vi "DSF.Engine.Transfer.Set Channel Blocks.vi"(10 "Block Descriptors":T1[](array[typedef]) {"count" format="%d elements"; "First Channel Descriptor"."base address" format="%016x"; "First Channel Descriptor"."Channel Parameters"."offset" format="%d bytes"}, 11 "Transfer in":refnum<class "DSF.Engine.Transfer.lvclass">) -> (3 "Transfer out":refnum<class "DSF.Engine.Transfer.lvclass">)   [LabVIEW 2017, in "DSF.Engine.lvlib" / "DSF.Engine.Transfer.lvclass"]
uses:
  DSF.Engine.Transfer.lvclass
  Shared/Typedefs/DSF.Shared.Typedefs.Configuration.Transfer.Channel Block Descriptor.ctl
  Shared/Typedefs/DSF.Shared.Typedefs.Configuration.Transfer.Channel Descriptor.ctl
  Shared/Typedefs/DSF.Shared.Typedefs.Configuration.Transfer.Channel Parameters.ctl
  Shared/Typedefs/DSF.Shared.Typedefs.Data Type.ctl
  DSF.Engine.Transfer.lvclass/DSF.Engine.Transfer.ctl
  DSF.Shared.lvlib
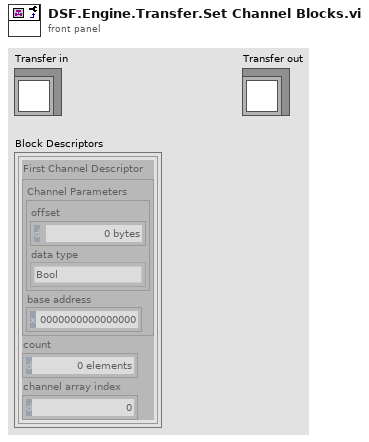
[diagram p1: front panel]
types:
  T1 = typedef "DSF.Shared.lvlib/DSF.Shared.Typedefs.Configuration.Transfer.Channel Block Descriptor.ctl" = cluster{"First Channel Descriptor":T2, "count":u64, "channel array index":u64}
  T2 = typedef "DSF.Shared.lvlib/DSF.Shared.Typedefs.Configuration.Transfer.Channel Descriptor.ctl" = cluster{"Channel Parameters":T3, "base address":u64}
  T3 = typedef "DSF.Shared.lvlib/DSF.Shared.Typedefs.Configuration.Transfer.Channel Parameters.ctl" = cluster{"offset":u64, "data type":T4}
  T4 = typedef "DSF.Shared.lvlib/DSF.Shared.Typedefs.Data Type.ctl" = enum8{"Bool", "SGL", "DBL", "I8", "I16", "I32", "I64", "U8", "U16", "U32", "U64"}
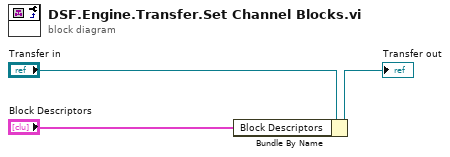
[diagram p0: block diagram]
diagram:
  n1 = Bundle By Name(cluster="Transfer in", "Block Descriptors"="Block Descriptors") -> (→"Transfer out":refnum<class "DSF.Engine.Transfer.lvclass">)
